vi "Create RPC Impl VI.vi"(8 "error in (no error)":errorcluster, 9 "String":string, 10 "LVClassLibrary Item in":refnum<vi>, 11 "Template VI in":refnum<vi>) -> (0 "error out":errorcluster, 2 "LVClassLibrary out":refnum<vi>, 3 "RPC Impl VI out":refnum<vi>)   [LabVIEW 2019, in "gRPC Template Creation Utility.lvlib"]
uses:
  gRPC Template Creation Utility.lvlib
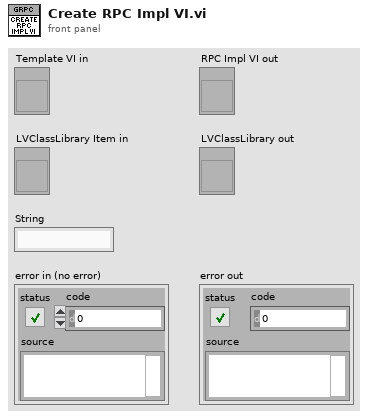
[diagram p1: front panel]
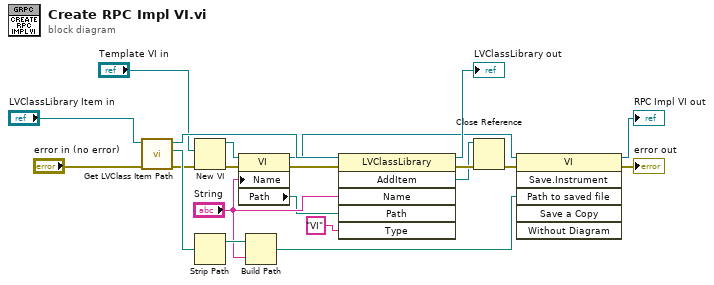
[diagram p0: block diagram]
diagram:
  n1 = call "Get LVClass Item Path.vi"("error in (no error)"="error in (no error)", "LVClassLibrary in"="LVClassLibrary Item in") -> ("error out"=w18:errorcluster, "Path"=w19:path, "LVClassLibrary out"=w21:refnum<vi>)  [unwired: 7 in]
  n2 = New VI(8:w18, 10:"Template VI in") -> (0:w10:errorcluster, 3:w6:refnum<vi>)  [unwired: 5 in]
  n3 = Strip Path(path=w19) -> (stripped path=w12:path)  [unwired: 1 out]
  n4 = property class="VI"(reference=w6, error in=w10, "Name"="String") -> (reference out=w7:refnum<vi>, error out=w2:errorcluster, "Path"=w9:path)
  n5 = Build Path(base path=w12, name or relative path="String") -> (appended path=w8:path)
  n6 = invoke class="LVClassLibrary" method="AddItem"(reference=w21, error in=w2, "Name"="String", "Path"=w9, "Type"="VI") -> (reference out=→"LVClassLibrary out":refnum<vi>, error out=w4:errorcluster, "AddItem"=w3:refnum<vi>)  [unwired: 1 in, 3 out]
  n7 = Close Reference(reference=w3, error in (no error)=w4) -> (error out=w5:errorcluster)
  n8 = invoke class="VI" method="Save.Instrument"(reference=w7, error in=w5, "Path to saved file"=w8) -> (reference out=→"RPC Impl VI out":refnum<vi>, error out=→"error out":errorcluster)  [unwired: 3 in, 4 out]
